vi "test2-LocalExternalStatusRegistrationViaAPI.vi"(8 "error in (no error)":errorcluster, 11 "TestCase in":refnum<class "testcase-CSMBroadcast.lvclass">) -> (0 "error out":errorcluster, 3 "TestCase out":refnum<class "testcase-CSMBroadcast.lvclass">)   [LabVIEW 2017, in "testcase-CSMBroadcast.lvclass"]
uses:
  testcase-CSMBroadcast.lvclass
  0b17d103-e67b-41be-a9eb-a2ee1311ff1f.vi
  5999693e-4f8a-4b34-ae87-f34dff5771be.vi
  52a2a10a-a04b-4bad-8df4-e1eb944f47cc.vi
  826f03dd-b4b5-4c6b-9085-8edf6da4f43b.vi
  src/user.lib/_NEVSTOP/Communicable State Machine(CSM)/AdvanceAPI/CSM - Get Module Attribute.vi
  <vilib>/addons/_JKI Toolkits/VI Tester/TestCase.llb/TestCase.lvclass
  src/user.lib/_NEVSTOP/Communicable State Machine(CSM)/Communicable State Machine.lvlib
  C:/Program Files (x86)/National Instruments/LabVIEW 2017/vi.lib/addons/_JKI Toolkits/VI Tester/TestCase.llb/TestCase.lvclass
panel:
  out "LoopCount 2":i32
  out "LoopCount":i32
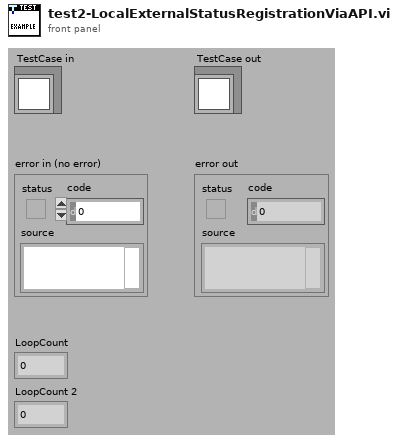
[diagram p1: front panel]
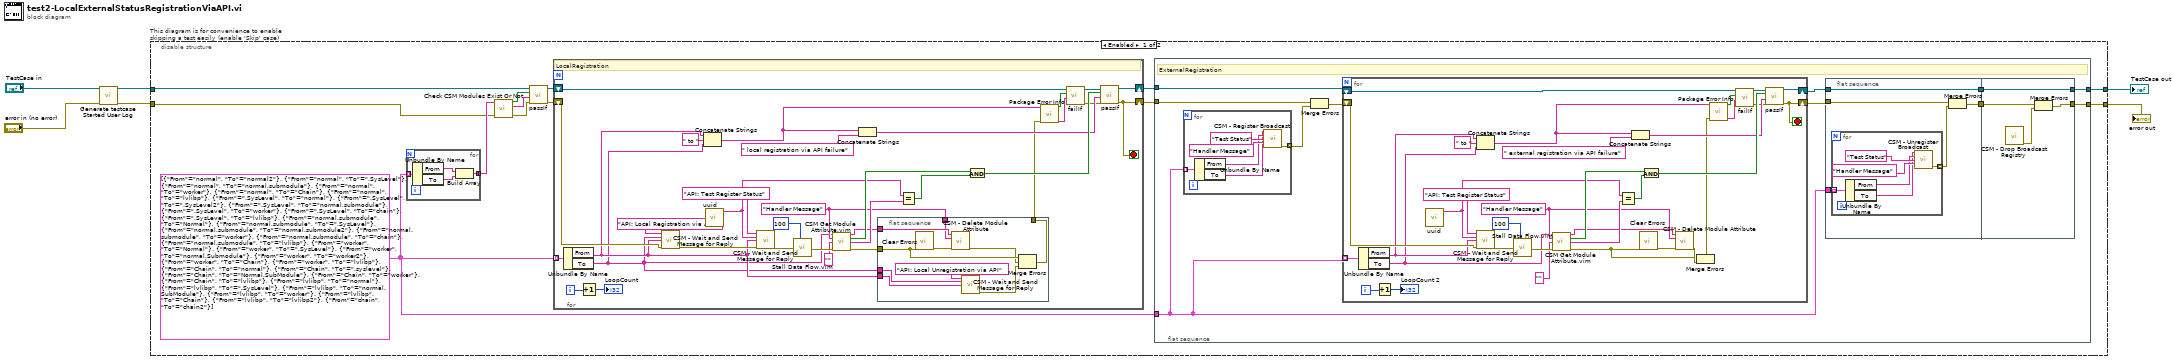
[diagram p0: block diagram]
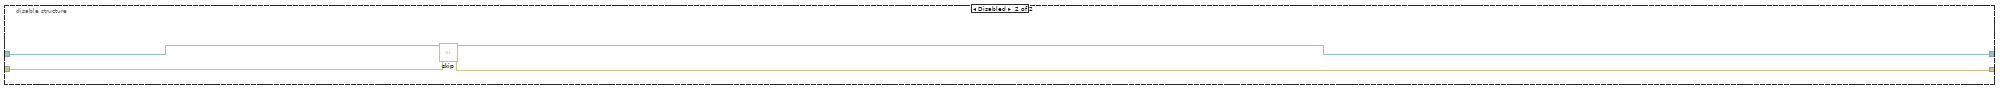
[diagram p2: hidden frame]
diagram:
  n1 = call "Generate testcase Started User Log.vi"("Error In"="error in (no error)") -> ("error out"=w1:errorcluster)  [unwired: 10 in]
  n2 = disable-structure "This diagram is for convenience to enable skipping a test easily (enable 'Skip' case)" shown="Enabled" {
    disable-tunnel: "TestCase in" -> [w12 w134]
    disable-tunnel: [w7 w132] -> w2
    disable-tunnel: [w6 w133] -> w4
    disable-tunnel: w1 -> [w10 w131]
    frame Enabled {
      w8 = cluster{"From":string, "To":string}[] [{"From"="normal", "To"="normal2"}, {"From"="normal", "To"=".SysLevel"}, {"From"="normal", "To"="normal.submodule"}, {"From"="normal", "To"="worker"}, {"From"="normal", "To"="Chain"}, {"From"="normal", "To"="lvlibp"}, {"From"=".SysLevel", "To"="normal"}, {"From"=".SysLevel", "To"=".SysLevel2"}, {"From"=".SysLevel", "To"="normal.submodule"}, {"From"=".SysLevel", "To"="worker"}, {"From"=".SysLevel", "To"="chain"}, {"From"=".SysLevel", "To"="lvlibp"}, {"From"="normal.submodule", "To"="Normal"}, {"From"="normal.submodule", "To"=".SysLevel"}, {"From"="normal.submodule", "To"="normal.submodule2"}, {"From"="normal.submodule", "To"="worker"}, {"From"="normal.submodule", "To"="chain"}, {"From"="normal.submodule", "To"="lvlibp"}, {"From"="worker", "To"="Normal"}, {"From"="worker", "To"=".SysLevel"}, {"From"="worker", "To"="normal.Submodule"}, {"From"="worker", "To"="worker2"}, {"From"="worker", "To"="Chain"}, {"From"="worker", "To"="lvlibp"}, {"From"="Chain", "To"="normal"}, {"From"="Chain", "To"=".syslevel"}, {"From"="Chain", "To"="Normal.SubModule"}, {"From"="Chain", "To"="worker"}, {"From"="Chain", "To"="lvlibp"}, {"From"="lvlibp", "To"="normal"}, {"From"="lvlibp", "To"=".SysLevel"}, {"From"="lvlibp", "To"="normal.SubModule"}, {"From"="lvlibp", "To"="worker"}, {"From"="lvlibp", "To"="Chain"}, {"From"="lvlibp", "To"="lvlibp2"}, {"From"="chain", "To"="chain2"}]
      n3 = for {
        tunnel: w8 -> [w22] mode=indexing
        tunnel: [w19] -> w15 mode=concatenating
        n4 = Unbundle By Name(w22) -> ("From"=w21:string, "To"=w20:string)
        n5 = Build Array(w21, w20) -> (w19:string[])
      }
      n6 = call "Check CSM Modules Exist Or Not.vi"("error in"=w10, "CSM names in"=w15) -> ("error out"=w13:errorcluster, "Debug string"=w14:string, "All Modules Exist?"=w16:bool)  [unwired: 7 in]
      n7 = call-dynamic "passIf.vi"("error in (no error)"=w13, "message (\"\")"=w14, "pass"=w16, "TestCase in"=w12) -> ("error out"=w9:errorcluster, "TestCase out"=w11:refnum<class "testcase-CSMBroadcast.lvclass">)  [unwired: 6 in]
      n8 = for {
        shift-right: [w35] -> w17
        shift-left: w9 -> [w36]
        shift-right: [w42] -> w18
        shift-left: w11 -> [w27]
        tunnel: w8 -> [w53] mode=indexing
        i -> [w55]
        stop <- w35 stop-if-true
        w37 = "Handler Message" ("To")
        # "LocalRegistration"
        n9 = Unbundle By Name(w53) -> ("From"=w32:string, "To"=w31:string)
        n10 = Increment(x=w55) -> (x+1=→"LoopCount":i32)
        n11 = call "CSM - Wait and Send Message for Reply.vi"("State"="API: Local Registration via API", "Arguments (\"\")"=w31, "Target Module"=w32, "Error In (No Error)"=w36) -> ("error out"=w50:errorcluster)  [unwired: 8 in, 3 out]
        n12 = Concatenate Strings(w32, " to " ("string"), w31) -> (w23:string)
        n13 = call "uuid.vi"() -> ("UUID"=w44:string)  [unwired: 11 in]
        n14 = call "CSM - Wait and Send Message for Reply.vi"("State"="API: Test Register Status", "Arguments (\"\")"=w44, "Target Module"=w32, "Error In (No Error)"=w50) -> ("error out"=w49:errorcluster)  [unwired: 8 in, 3 out]
        n15 = call "Stall Data Flow.vim"("value in"=w49, "milliseconds to wait"=u32 100) -> ("value out"=w47:errorcluster)  [unwired: 1 out]
        n16 = call "CSM Get Module Attribute.vim"("CSM Name"=w31, "Attribute"=w37, "Default Value (Empty Variant)"="", "Error In"=w47) -> ("CSM Name (Dup)"=w38:string, "Found"=w46:bool, "Value"=w43:string, "error out"=w39:errorcluster)  [unwired: 7 in, 1 out]
        n17 = Concatenate Strings(w23, " local registration via API failure" ("string")) -> (w30:string)
        n18 = flat-sequence {
          tunnel: w39 -> [w59]
          tunnel: w38 -> [w64]
          tunnel: w37 -> [w63]
          tunnel: w31 -> [w61]
          tunnel: w32 -> [w60]
          tunnel: [w56] -> _
          tunnel: [w56] -> w24
          frame #0 {
            n19 = call <vilib>:"Clear Errors.vi"("error in (no error)"=w59) -> ("error out"=w65:errorcluster)  [unwired: 5 in, 1 out]
            n20 = call "CSM - Delete Module Attribute.vi"("CSM Name"=w64, "Attribute"=w63, "Error In"=w65) -> ("error out"=w58:errorcluster)  [unwired: 9 in, 3 out]
            n21 = call "CSM - Wait and Send Message for Reply.vi"("State"="API: Local Unregistration via API", "Arguments (\"\")"=w61, "Target Module"=w60) -> ("error out"=w57:errorcluster)  [unwired: 9 in, 3 out]
            n22 = Merge Errors(w59, w58, w57) -> (w56:errorcluster)
          }
        }
        n23 = Equal?(x=w44, y=w43) -> (x = y?=w41:bool)
        n24 = And(x=w46, y=w41) -> (x .and. y?=w40:bool)
        n25 = call "Package Error Info.vi"("error in"=w24, "String in"=w23) -> ("packed error info out"=w28:string, "error status"=w29:bool)  [unwired: 8 in]
        n26 = call-dynamic "failIf.vi"("message (\"\")"=w28, "fail"=w29, "TestCase in"=w27) -> ("error out"=w25:errorcluster, "TestCase out"=w26:refnum<class "testcase-CSMBroadcast.lvclass">)  [unwired: 7 in]
        n27 = call-dynamic "passIf.vi"("error in (no error)"=w25, "message (\"\")"=w30, "pass"=w40, "TestCase in"=w26) -> ("error out"=w35:errorcluster, "TestCase out"=w42:refnum<class "testcase-CSMBroadcast.lvclass">)  [unwired: 6 in]
      }
      n28 = flat-sequence {
        tunnel: w18 -> [w76]
        tunnel: w17 -> [w74]
        tunnel: w8 -> [w73]
        tunnel: [w67] -> w7
        tunnel: [w66] -> w6
        frame #0 {
          # "ExternalRegistration"
          n29 = for {
            tunnel: w73 -> [w97] mode=indexing
            tunnel: [w92] -> w72 mode=indexing
            n30 = Unbundle By Name(w97) -> ("From"=w94:string, "To"=w93:string)
            n31 = call "CSM - Register Broadcast.vi"("CSM Name(Empty for Broadcast Event)"=w93, "Source CSM Name (* as Default)"=w94, "Trigger"="Test Status" ("Status"), "API (If \"\", Same as Trigger)"="Handler Message" ("Response Message (If \"\", Same as Source Message)")) -> ("error out"=w92:errorcluster)  [unwired: 10 in, 1 out]
          }
          n32 = Merge Errors(w74, w72) -> (w75:errorcluster)
          n33 = for {
            shift-right: [w112] -> w71
            shift-left: w75 -> [w113]
            shift-right: [w119] -> w70
            shift-left: w76 -> [w102]
            tunnel: w73 -> [w128] mode=indexing
            i -> [w130]
            stop <- w112 stop-if-true
            w114 = "Handler Message" ("To")
            n34 = Unbundle By Name(w128) -> ("From"=w107:string, "To"=w106:string)
            n35 = Increment(x=w130) -> (x+1=→"LoopCount 2":i32)
            n36 = call "uuid.vi"() -> ("UUID"=w121:string)  [unwired: 11 in]
            n37 = Concatenate Strings(w107, " to " ("string"), w106) -> (w98:string)
            n38 = call "CSM - Wait and Send Message for Reply.vi"("State"="API: Test Register Status", "Arguments (\"\")"=w121, "Target Module"=w107, "Error In (No Error)"=w113) -> ("error out"=w126:errorcluster)  [unwired: 8 in, 3 out]
            n39 = call "Stall Data Flow.vim"("value in"=w126, "milliseconds to wait"=u32 100) -> ("value out"=w124:errorcluster)  [unwired: 1 out]
            n40 = call "CSM Get Module Attribute.vim"("CSM Name"=w106, "Attribute"=w114, "Default Value (Empty Variant)"="", "Error In"=w124) -> ("CSM Name (Dup)"=w115:string, "Found"=w123:bool, "Value"=w120:string, "error out"=w110:errorcluster)  [unwired: 7 in, 1 out]
            n41 = Equal?(x=w121, y=w120) -> (x = y?=w118:bool)
            n42 = Concatenate Strings(w98, " external registration via API failure" ("string")) -> (w105:string)
            n43 = call <vilib>:"Clear Errors.vi"("error in (no error)"=w110) -> ("error out"=w116:errorcluster)  [unwired: 5 in, 1 out]
            n44 = And(x=w123, y=w118) -> (x .and. y?=w117:bool)
            n45 = call "CSM - Delete Module Attribute.vi"("CSM Name"=w115, "Attribute"=w114, "Error In"=w116) -> ("error out"=w111:errorcluster)  [unwired: 9 in, 3 out]
            n46 = Merge Errors(w110, w111) -> (w99:errorcluster)
            n47 = call "Package Error Info.vi"("error in"=w99, "String in"=w98) -> ("packed error info out"=w103:string, "error status"=w104:bool)  [unwired: 8 in]
            n48 = call-dynamic "failIf.vi"("message (\"\")"=w103, "fail"=w104, "TestCase in"=w102) -> ("error out"=w100:errorcluster, "TestCase out"=w101:refnum<class "testcase-CSMBroadcast.lvclass">)  [unwired: 7 in]
            n49 = call-dynamic "passIf.vi"("error in (no error)"=w100, "message (\"\")"=w105, "pass"=w117, "TestCase in"=w101) -> ("error out"=w112:errorcluster, "TestCase out"=w119:refnum<class "testcase-CSMBroadcast.lvclass">)  [unwired: 6 in]
          }
          n50 = flat-sequence {
            tunnel: w73 -> [w81]
            tunnel: w71 -> [w79]
            tunnel: w70 -> [w80]
            tunnel: [w80] -> w69
            tunnel: [w77] -> w68
            tunnel: [w89] -> w66
            tunnel: [w91] -> w67
            tunnel: w69 -> [w91]
            tunnel: w68 -> [w90]
            frame #0 {
              n51 = for {
                tunnel: w81 -> [w87] mode=indexing
                tunnel: [w82] -> w78 mode=indexing
                n52 = Unbundle By Name(w87) -> ("From"=w84:string, "To"=w83:string)
                n53 = call "CSM - Unregister Broadcast.vi"("CSM Name(Empty for Broadcast Event)"=w83, "Source CSM Name (* as Default)"=w84, "Trigger"="Test Status" ("Status"), "API (\"*\" as Default)"="Handler Message" ("Response Message (If \"\", Same as Source Message)")) -> ("error out"=w82:errorcluster)  [unwired: 10 in, 1 out]
              }
              n54 = Merge Errors(w79, w78) -> (w77:errorcluster)
            }
            frame #1 {
              n55 = call "CSM - Drop Broadcast Registry.vi"() -> ("error out"=w88:errorcluster)  [unwired: 15 in]
              n56 = Merge Errors(w90, w88) -> (w89:errorcluster)
            }
          }
        }
      }
    }
    frame Disabled {
      # "skip test result while test is under development"
      n57 = call <vilib>:"skip.vi"("error in (no error)"=w131, "TestCase in"=w134) -> ("error out"=w133:errorcluster, "TestCase out"=w132:refnum<class "testcase-CSMBroadcast.lvclass">)  [unwired: 8 in]
    }
  }
  "error out" <- w4
  "TestCase out" <- w2
